vi "Application Mode.vi"(8 "error in (no error)":errorcluster) -> (0 "error out":errorcluster, 3 "Run Time Mode?":bool)   [LabVIEW 2014]
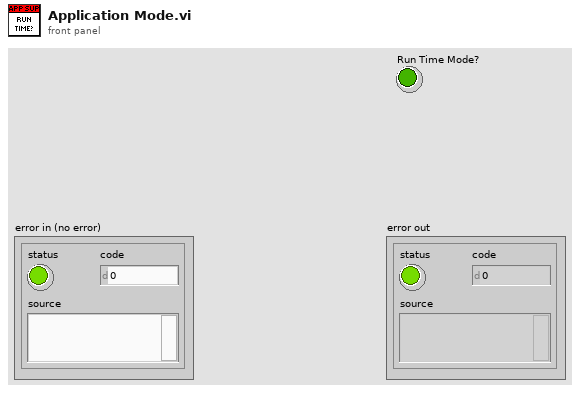
[diagram p1: front panel]
types:
  T1 = enum32{"invalid app kind", "Development System", "Run Time System", "Student Edition", "Embedded LabVIEW", "Evaluation", "Custom"}
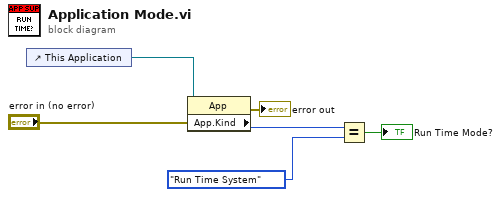
[diagram p0: block diagram]
diagram:
  n1 = control-ref of="This Application"() -> (w6:refnum<vi>)
  n2 = property class="App"(reference=w6, error in="error in (no error)") -> (error out=→"error out":errorcluster, "App.Kind"=w3:T1)  [unwired: 1 out]
  n3 = Equal?(x=w3, y=T1."Run Time System" ("Application:Kind")) -> (x = y?=→"Run Time Mode?":bool)
